vi "Extended User Data.vi"(7 "Action (0 : Read Data)":i32(ring) items=["Read Data", "Write Data", "Clear Data", "Clear All Data"], 8 "error in (no error)":errorcluster, 10 "User Data In":T1 {"Model" items=["DX100/DX200", "DX1000/DX2000"]}, 11 "VISA resource name":refnum<visa-resource-name>) -> (0 "error out":errorcluster, 1 "Model":i32(ring) items=["DX100/DX200", "DX1000/DX2000"], 2 "User Data Out":T1 {"Model" items=["DX100/DX200", "DX1000/DX2000"]}, 3 "VISA resource name out":refnum<visa-resource-name>)   [LabVIEW 2011, in "Yokogawa DX Series.lvlib"]
doc: "Writes, reads, and clears data of the type User Data In to the connected VISA session."
uses:
  <instrlib>/Yokogawa DX Series/Yokogawa DX Series.lvlib
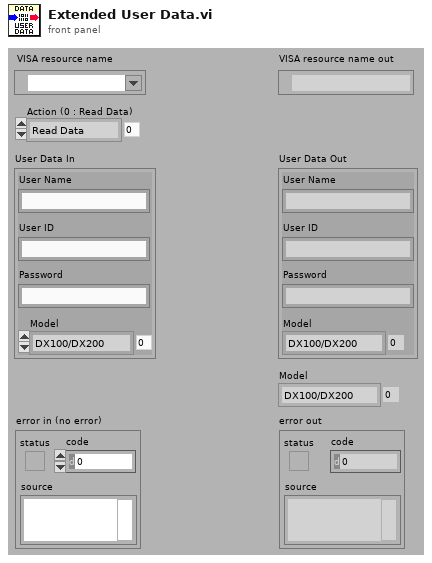
[diagram p1: front panel]
types:
  T1 = cluster{"User Name":string, "User ID":string, "Password":string, "Model":i32}
  T2 = cluster{"User Name":string, "User ID":string, "Password":string, "Model":u16}[]
  T3 = cluster{"User Name":string, "User ID":string, "Password":string, "Model":i32}[]
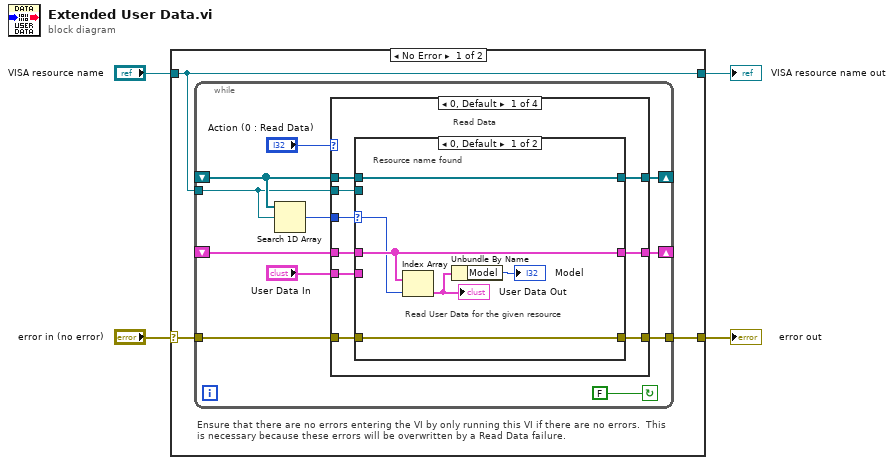
[diagram p0: block diagram]
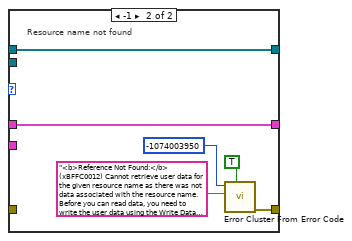
[diagram p2: hidden frame]
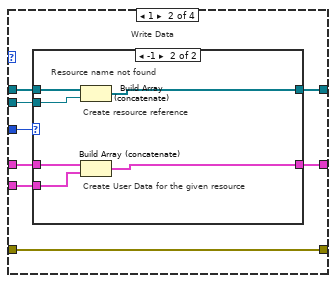
[diagram p3: hidden frame]
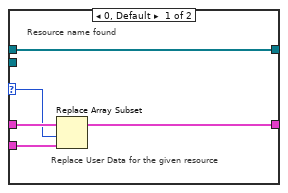
[diagram p4: hidden frame]
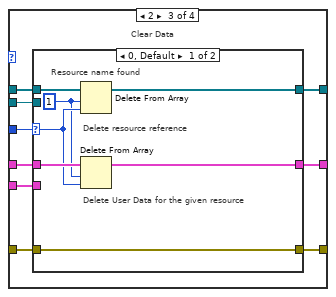
[diagram p5: hidden frame]
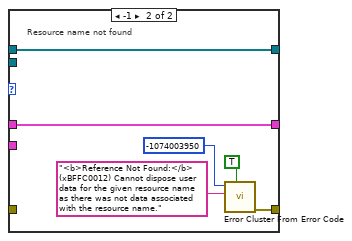
[diagram p6: hidden frame]
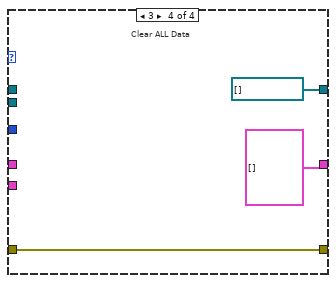
[diagram p7: hidden frame]
diagram:
  n1 = case shown="No Error" "error in (no error)" {
    selector: "error in (no error)" -> [w5 w84]
    tunnel: [w7 w85] -> w3
    tunnel: "VISA resource name" -> [w7 w85]
    tunnel: [w6 w84] -> w1
    frame No Error {
      # "Ensure that there are no errors entering the VI by only running this VI if there are no errors.  This is necessary because these errors will be overwritten by a Read Data failure."
      n2 = while {
        shift-right: [w17] -> _
        shift-left: _ -> [w16]
        shift-right: [w12] -> _
        shift-left: _ -> [w13]
        tunnel: w7 -> [w15]
        tunnel: [w10] -> w6
        tunnel: w5 -> [w9]
        stop <- FALSE continue-if-true
        n3 = Search 1D Array(1D array=w16, element=w15) -> (index of element=w14:i32)  [unwired: 1 out]
        n4 = case shown="0, Default" "Action (0 : Read Data)" {
          tunnel: [w27 w42 w63 refnum<visa-resource-name>[] []] -> w17
          tunnel: w16 -> [w26 w41 w62 _]
          tunnel: w15 -> [w25 w40 w61 _]
          tunnel: w14 -> [w24 w47 w67 _]
          tunnel: w13 -> [w23 w46 w66 _]
          tunnel: [w22 w44 w64 T2 []] -> w12
          tunnel: "User Data In" -> [w21 w45 w65 _]
          tunnel: [w20 w43 w60 w83] -> w10
          tunnel: w9 -> [w19 w43 w59 w83]
          frame 0, Default {
            # "Read Data"
            n5 = case shown="0, Default" w24 {
              selector: w24 -> [w31 _]
              tunnel: [w33 w39] -> w27
              tunnel: w26 -> [w33 w39]
              tunnel: w25 -> [_ _]
              tunnel: w23 -> [w32 w38]
              tunnel: [w32 w38] -> w22
              tunnel: w21 -> [_ _]
              tunnel: [w30 w34] -> w20
              tunnel: w19 -> [w30 _]
              frame 0, Default {
                # "Read User Data for the given resource"
                # "Resource name found"
                n6 = Index Array(array=w32, index=w31) -> (element=w29:T1)
                "User Data Out" <- w29
                n7 = Unbundle By Name(w29) -> ("Model"=→"Model":i32)
              }
              frame -1 {
                # "Resource name not found"
                n8 = call <vilib>:"Error Cluster From Error Code.vi"("show call chain? (False)"=TRUE, "error message (\"\")"="<b>Reference Not Found:</b>  (xBFFC0012) Cannot retrieve user data for the given resource name as there was not data associated with the resource name.  Before you can read data, you need to write the user data using the Write Data action of this User Data VI. ", "error code (0)"=-1074003950) -> ("error out"=w34:errorcluster)  [unwired: 1 in, 5 out]
              }
            }
          }
          frame 1 {
            # "Write Data"
            n9 = case shown="-1" w47 {
              selector: w47 -> [w51 _]
              tunnel: w46 -> [w52 w55]
              tunnel: w45 -> [w50 w54]
              tunnel: [w49 w53] -> w44
              tunnel: [w48 w56] -> w42
              tunnel: w41 -> [w48 w58]
              tunnel: w40 -> [_ w57]
              frame 0, Default {
                # "Replace User Data for the given resource"
                # "Resource name found"
                n10 = Replace Array Subset(array=w52, new element=w50, index=w51) -> (w49:T3)
              }
              frame -1 {
                # "Create User Data for the given resource"
                # "Create resource reference"
                # "Resource name not found"
                n11 = Build Array (concatenate)(w58, w57) -> (w56:refnum<visa-resource-name>[])
                n12 = Build Array (concatenate)(w55, w54) -> (w53:T3)
              }
            }
          }
          frame 2 {
            # "Clear Data"
            n13 = case shown="0, Default" w67 {
              selector: w67 -> [w72 _]
              tunnel: w66 -> [w74 w79]
              tunnel: w65 -> [_ _]
              tunnel: [w73 w79] -> w64
              tunnel: [w69 w80] -> w63
              tunnel: w62 -> [w70 w80]
              tunnel: w61 -> [_ _]
              tunnel: [w68 w75] -> w60
              tunnel: w59 -> [w68 _]
              frame 0, Default {
                w71 = 1
                # "Delete User Data for the given resource"
                # "Delete resource reference"
                # "Resource name found"
                n14 = Delete From Array(array=w70, length=w71, index=w72) -> (array with subset deleted=w69:refnum<visa-resource-name>[])  [unwired: 1 out]
                n15 = Delete From Array(array=w74, length=w71, index=w72) -> (array with subset deleted=w73:T3)  [unwired: 1 out]
              }
              frame -1 {
                # "Resource name not found"
                n16 = call <vilib>:"Error Cluster From Error Code.vi"("show call chain? (False)"=TRUE, "error message (\"\")"="<b>Reference Not Found:</b>  (xBFFC0012) Cannot dispose user data for the given resource name as there was not data associated with the resource name.", "error code (0)"=-1074003950) -> ("error out"=w75:errorcluster)  [unwired: 1 in, 5 out]
              }
            }
          }
          frame 3 {
            # "Clear ALL Data"
          }
        }
      }
    }
    frame Error {
    }
  }
  "VISA resource name out" <- w3
  "error out" <- w1
